vi "PH_VacuumControl.ProcPeriodic.vi"(0 "i ref in":refnum<vi>, 3 "ms timeout (100)":i32=100, 5 "error in (no error)":errorcluster) -> (14 "i ref out":refnum<vi>, 17 "timed out":bool, 19 "error out":errorcluster)   [LabVIEW 2014, in "PH_VacuumControl.lvlib"]
doc: "This method serves to periodically do things like reading values from the HW. Methods that should be executed periodically should be called from THIS methode. Add code here."
uses:
  PH_VacuumControl.lvlib
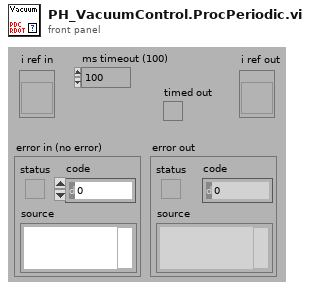
[diagram p1: front panel]
types:
  T1 = typedef "PH_VacuumControl.lvlib/PH_VacuumControl.i attribute.ctl" = cluster{"GUI Refs":cluster{"Exit":refnum<vi>, "Set Unit":refnum<vi>, "Device found":refnum<vi>, "Busy":refnum<vi>, "State":refnum<vi>, "Delete":refnum<vi>, "Channels":refnum<vi>, "Channel Name":refnum<vi>, "Trend":refnum<vi>, "Logarithmic":refnum<vi>, "Limit reached":refnum<vi>, "Channel Name 1 MT":refnum<vi>, "Channel Name 2 MT":refnum<vi>, "Trend MT":refnum<vi>, "Logarithmic MT":refnum<vi>, "Limit reached MT":refnum<vi>}, "Device found":bool, "Busy":bool, "Selected Unit":i32, "Channels [mbar]":T2, "Channel Names":cluster{"Channel 1":string, "Channel 2":string, "Channel 3":string, "Channel 4":string, "Channel 5":string, "Channel 6":string}, "Status":T3, "AGCxxx VISA Cluster":T4, "Instr Firmware Revision":string, "Service IDs Pressure":cluster{"Channel 1":i32, "Channel 2":i32, "Channel 3":i32, "Channel 4":i32, "Channel 5":i32, "Channel 6":i32}, "Service IDs Limits":cluster{"Channel 1":i32, "Channel 2":i32, "Channel 3":i32, "Channel 4":i32, "Channel 5":i32, "Channel 6":i32}, "Trend":cluster{"Start Point":timestamp, "Pressures [mbar] Channel 1":dbl[], "Pressures [mbar] Channel 2":dbl[], "Pressures [mbar] Channel 3":dbl[], "Pressures [mbar] Channel 4":dbl[], "Pressures [mbar] Channel 5":dbl[], "Pressures [mbar] Channel 6":dbl[], "Timebase [s]":i32[], "Trend Channel":u16, "Start Fit":dbl, "Trend Channel 1 MT":u16, "Trend Channel 2 MT":u16, "Start or continue Fit MT":dbl, "Continue or start Fit MT":dbl, "Datasets strored":i32, "Dataarray Size":i32}, "Running":bool}
  T2 = typedef "PH_VacuumControl.lvlib/PH_VacuumControl.Channels.ctl" = cluster{"Channel 1":dbl, "Channel 2":dbl, "Channel 3":dbl, "Channel 4":dbl, "Channel 5":dbl, "Channel 6":dbl, "Name Channel 1":string, "Name Channel 2":string, "Name Channel 3":string, "Name Channel 4":string, "Name Channel 5":string, "Name Channel 6":string, "Upper Limit":dbl, "Upper Limit 2":dbl, "Upper Limit 3":dbl, "Upper Limit 4":dbl, "Upper Limit 5":dbl, "Upper Limit 6":dbl}
  T3 = typedef "PH_StatusHandler.lvlib/PH_StatusHandler.Status.ctl" = i16
  T4 = typedef "AGCxxx - Driver.lvlib/AGCxxx VISA Control.ctl" = cluster{"VISA resource name":refnum<visa-resource-name>, "VISA Timeout Value (1000 ms)":u32, "Lock Timeout (1000 ms)":u32, "MAX Channel (6)":i32}
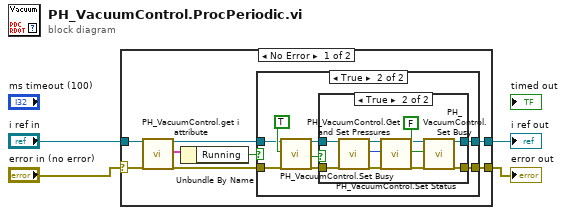
[diagram p0: block diagram]
diagram:
  n1 = case shown="No Error" "error in (no error)" {
    selector: "error in (no error)" -> [w10 w36]
    tunnel: "i ref in" -> [w8 w35]
    tunnel: [w12 w36] -> w4
    tunnel: [w11 w35] -> w3
    frame No Error {
      n2 = call "PH_VacuumControl.get i attribute.vi"("i ref in"=w8, "error in (no error)"=w10) -> ("i ref out"=w7:refnum<vi>, "i attribute"=w6:T1, "error out"=w9:errorcluster)  [unwired: 15 in]
      n3 = Unbundle By Name(w6) -> ("Running"=w5:bool)
      n4 = case shown="True" w5 {
        tunnel: [w13 w20] -> w12
        tunnel: [w14 w19] -> w11
        tunnel: w9 -> [w13 w16]
        tunnel: w7 -> [w14 w15]
        frame False {
        }
        frame True {
          n5 = call "PH_VacuumControl.Set Busy.vi"("i ref in"=w15, "Busy"=TRUE, "error in (no error)"=w16) -> ("i ref out"=w21:refnum<vi>, "changed"=w17:bool, "error out"=w22:errorcluster)  [unwired: 14 in]
          n6 = case shown="True" w17 {
            tunnel: w22 -> [w23 w34]
            tunnel: w21 -> [w24 w33]
            tunnel: [w23 w32] -> w20
            tunnel: [w24 w31] -> w19
            frame False {
            }
            frame True {
              n7 = call "PH_VacuumControl.Get and Set Pressures.vi"("i ref in"=w33, "error in (no error)"=w34) -> ("i ref out"=w29:refnum<vi>, "Status"=w27:T3, "error out"=w28:errorcluster)  [unwired: 15 in]
              n8 = call "PH_VacuumControl.Set Status.vi"("i ref in"=w29, "Status"=w27, "error in (no error)"=w28) -> ("i ref out"=w26:refnum<vi>, "error out"=w25:errorcluster)  [unwired: 15 in]
              n9 = call "PH_VacuumControl.Set Busy.vi"("i ref in"=w26, "Busy"=FALSE, "error in (no error)"=w25) -> ("i ref out"=w31:refnum<vi>, "error out"=w32:errorcluster)  [unwired: 14 in, 1 out]
            }
          }
        }
      }
    }
    frame Error {
    }
  }
  "error out" <- w4
  "i ref out" <- w3
